vi "Dot.vi"(9 "Points Ajustés":dbl[](array[numeric]), 10 "Y":dbl[](array[numeric])) -> (2 "dot(X,Y)":dbl)   [LabVIEW 2012]
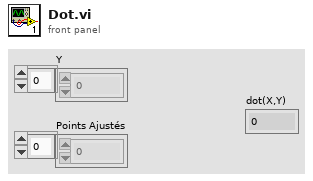
[diagram p1: front panel]
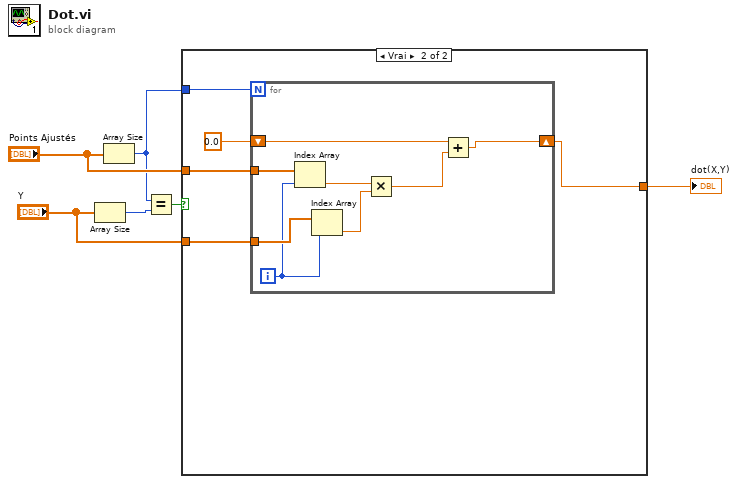
[diagram p0: block diagram]
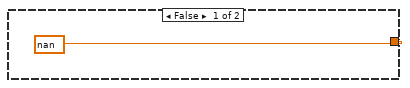
[diagram p2: hidden frame]
diagram:
  n1 = Array Size(array="Y") -> (size(s)=w3:i32)
  n2 = Array Size(array="Points Ajustés") -> (size(s)=w4:i32)
  n3 = Equal?(x=w4, y=w3) -> (x = y?=w2:bool)
  n4 = case shown="Vrai" w2 {
    tunnel: w4 -> [_ w12]
    tunnel: "Points Ajustés" -> [_ w10]
    tunnel: "Y" -> [_ w9]
    tunnel: [nan w8] -> w1
    frame False {
    }
    frame True {
      n5 = for {
        N: w12 -> [_]
        shift-right: [w18] -> w8
        shift-left: 0.0 -> [w20]
        tunnel: w10 -> [w15]
        tunnel: w9 -> [w14]
        i -> [w13]
        n6 = Index Array(array=w15, index=w13) -> (element=w17:dbl)
        n7 = Index Array(array=w14, index=w13) -> (element=w16:dbl)
        n8 = Multiply(x=w17, y=w16) -> (x*y=w19:dbl)
        n9 = Add(x=w20, y=w19) -> (x+y=w18:dbl)
      }
    }
  }
  "dot(X,Y)" <- w1
